vi "RF627_EXAMPLE.vi"() -> ()   [LabVIEW 2019]
doc: "This example VI calls the .NET DLL that accompanies it, which is a .NET class built in C# to emulate a very basic calculator."
uses:
  C:/Users/aagolovachev/Desktop/RLD_T14_2dScan/src/RF62X/RF62X-SDK/examples/LabVIEW/rf62Xsdk.dll
  rf62Xsdk.dll
panel:
  out "xemr":u16
  out "zmr":u16
  out "ReadParams":bool
  in  "index":i32
  in  "protocol":i32(ring)=1 items=["SERVICE_PROTOKOL"=1, "ETHERNET_IP"=2, "MODBUS_TCP"=3]
  out "Connect 2":bool
  in  "?":bool
  out "Connect":bool
  out "Count Points":i32
  out "XY Graph":cluster{"X":sgl, "Z":sgl}[](graph)
  out "Count":i32
  out "SdkInit":bool
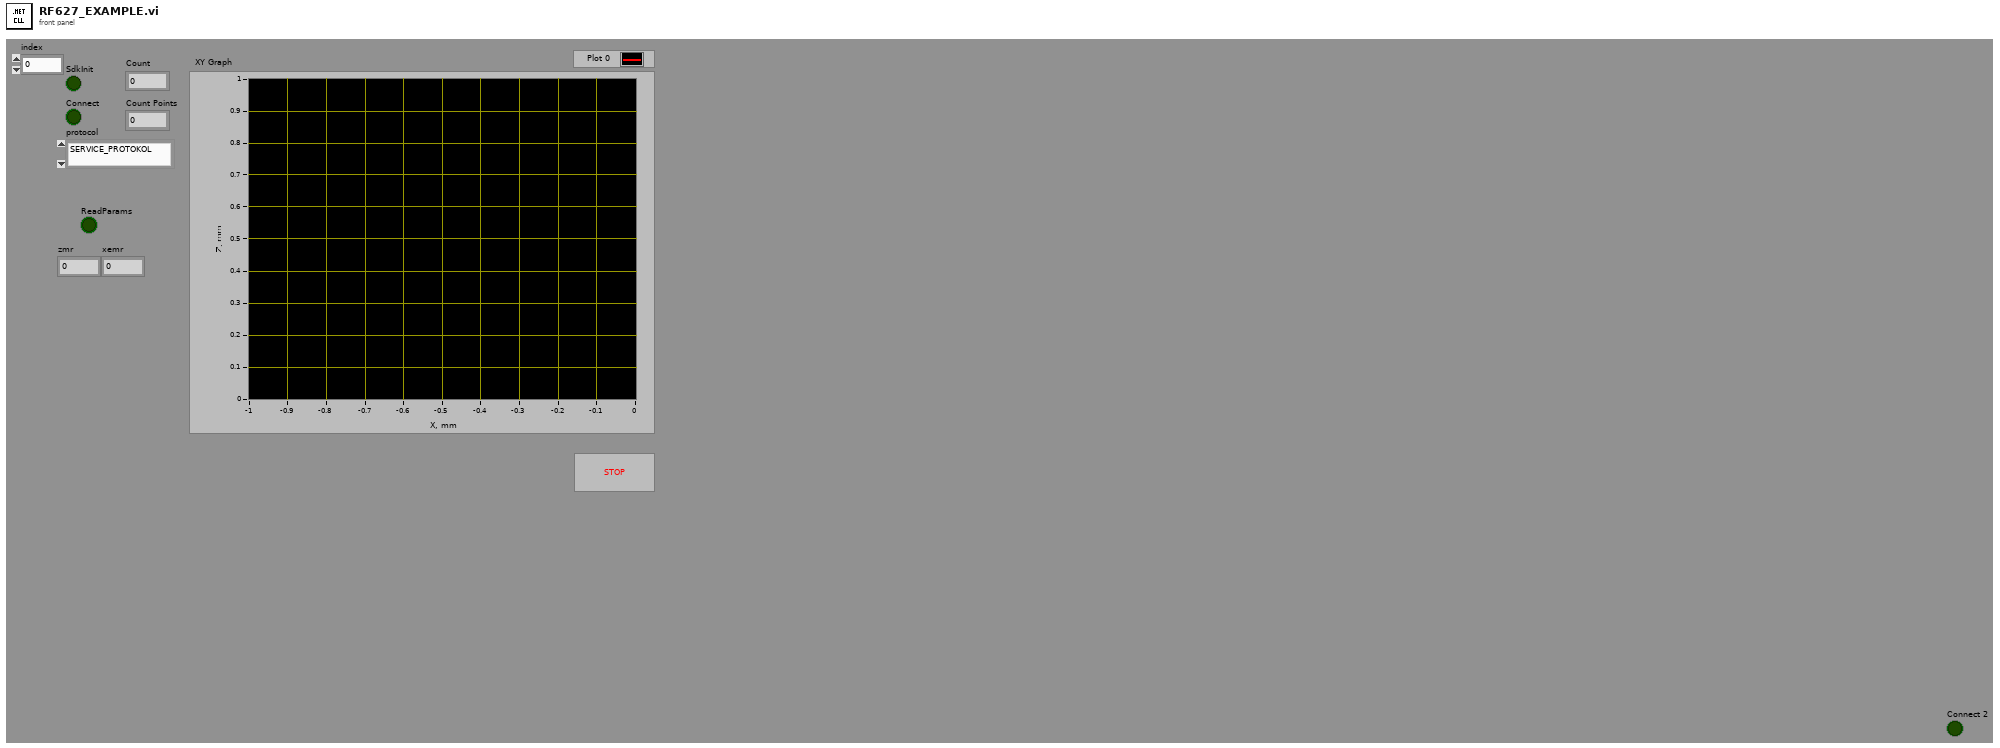
[diagram p1: front panel]
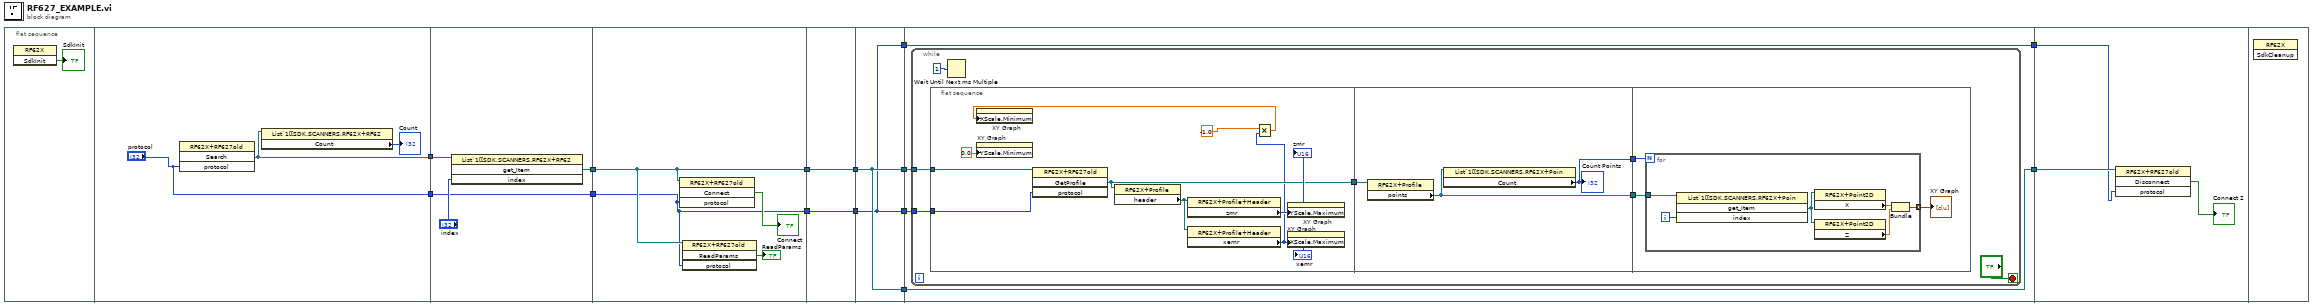
[diagram p0: block diagram]
diagram:
  n1 = flat-sequence {
    tunnel: [w17] -> w12
    tunnel: ["protocol"] -> w6
    tunnel: [w21] -> w14
    tunnel: w12 -> [w20]
    tunnel: [w19] -> w7
    tunnel: w6 -> [w19]
    tunnel: w14 -> [w25]
    tunnel: [w25] -> w13
    tunnel: w7 -> [w24]
    tunnel: [w24] -> w5
    tunnel: w13 -> [w28]
    tunnel: [w28] -> w10
    tunnel: w5 -> [w27]
    tunnel: [w27] -> w4
    tunnel: [w30] -> w11
    tunnel: w10 -> [w30]
    tunnel: [w30] -> w8
    tunnel: w4 -> [w29]
    tunnel: [w29] -> w3
    tunnel: [w29] -> w1
    tunnel: w11 -> [w34]
    tunnel: [w33] -> w9
    tunnel: w8 -> [w33]
    tunnel: w3 -> [w32]
    tunnel: [w31] -> w2
    tunnel: w1 -> [w31]
    tunnel: w9 -> [w64]
    tunnel: w2 -> [w63]
    frame #0 {
      n2 = invoke class="RF62X" method="SdkInit"() -> ("SdkInit"=→"SdkInit":bool)  [unwired: 3 in, 2 out]
    }
    frame #1 {
      n3 = invoke class="RF62X+RF627old" method="Search"("protocol"="protocol") -> ("Search"=w17:refnum<k24>)  [unwired: 3 in, 3 out]
      n4 = property class="List`1[[SDK.SCANNERS.RF62X+RF62"(reference=w17) -> ("Count"=→"Count":i32)  [unwired: 1 in, 2 out]
    }
    frame #2 {
      n5 = invoke class="List`1[[SDK.SCANNERS.RF62X+RF62" method="get_Item"(reference=w20, "index"="index") -> ("get_Item"=w21:refnum<k24>)  [unwired: 2 in, 3 out]
    }
    frame #3 {
      n6 = invoke class="RF62X+RF627old" method="Connect"(reference=w25, "protocol"=w24) -> ("Connect"=→"Connect":bool)  [unwired: 2 in, 3 out]
      n7 = invoke class="RF62X+RF627old" method="ReadParams"(reference=w25, "protocol"=w24) -> ("ReadParams"=→"ReadParams":bool)  [unwired: 2 in, 3 out]
    }
    frame #4 {
    }
    frame #5 {
    }
    frame #6 {
      n8 = while {
        tunnel: w34 -> [w39]
        tunnel: w32 -> [w35]
        stop <- "?" stop-if-true
        n9 = flat-sequence {
          tunnel: w39 -> [w50]
          tunnel: [w47] -> w38
          tunnel: w35 -> [w42]
          tunnel: w38 -> [w53]
          tunnel: [w52] -> w37
          tunnel: [w51] -> w36
          tunnel: w37 -> [w55]
          tunnel: w36 -> [w54]
          frame #0 {
            n10 = property on="XY Graph" class="XYGraph (strict)"("YScale.Minimum"=0.0 ("Y Scale.Range:Minimum")) -> ()  [unwired: 2 in, 2 out]
            n11 = invoke class="RF62X+RF627old" method="GetProfile"(reference=w50, "protocol"=w42) -> ("GetProfile"=w47:refnum<k24>)  [unwired: 2 in, 3 out]
            n12 = property class="RF62X+Profile"(reference=w47) -> ("header"=w48:refnum<k24>)  [unwired: 1 in, 2 out]
            n13 = property class="RF62X+Profile+Header"(reference=w48) -> ("zmr"=w49:u16)  [unwired: 1 in, 2 out]
            "zmr" <- w49
            n14 = property class="RF62X+Profile+Header"(reference=w48) -> ("xemr"=w44:u16)  [unwired: 1 in, 2 out]
            "xemr" <- w44
            n15 = Multiply(x=-1.0 ("Y Scale.Range:Minimum"), y=w44) -> (x*y=w43:dbl)
            n16 = property on="XY Graph" class="XYGraph (strict)"("XScale.Minimum"=w43) -> ()  [unwired: 2 in, 2 out]
            n17 = property on="XY Graph" class="XYGraph (strict)"("YScale.Maximum"=w49) -> ()  [unwired: 2 in, 2 out]
            n18 = property on="XY Graph" class="XYGraph (strict)"("XScale.Maximum"=w44) -> ()  [unwired: 2 in, 2 out]
          }
          frame #1 {
            n19 = property class="RF62X+Profile"(reference=w53) -> ("points"=w52:refnum<k24>)  [unwired: 1 in, 2 out]
            n20 = property class="List`1[[SDK.SCANNERS.RF62X+Poin"(reference=w52) -> ("Count"=w51:i32)  [unwired: 1 in, 2 out]
            "Count Points" <- w51
          }
          frame #2 {
            n21 = for {
              N: w54 -> [_]
              tunnel: [w61] -> w56 mode=indexing
              tunnel: w55 -> [w57]
              i -> [w62]
              n22 = invoke class="List`1[[SDK.SCANNERS.RF62X+Poin" method="get_Item"(reference=w57, "index"=w62) -> ("get_Item"=w60:refnum<k24>)  [unwired: 2 in, 3 out]
              n23 = property class="RF62X+Point2D"(reference=w60) -> ("X"=w59:sgl)  [unwired: 1 in, 2 out]
              n24 = property class="RF62X+Point2D"(reference=w60) -> ("Z"=w58:sgl)  [unwired: 1 in, 2 out]
              n25 = Bundle("X"=w59, "Z"=w58) -> (w61:cluster{"X":sgl, "Z":sgl})  [unwired: 1 in]
            }
            "XY Graph" <- w56
          }
        }
        n26 = Wait Until Next ms Multiple(millisecond multiple=u32 1 ("millisecond timer value")) -> ()  [unwired: 1 out]
      }
    }
    frame #7 {
      n27 = invoke class="RF62X+RF627old" method="Disconnect"(reference=w64, "protocol"=w63) -> ("Disconnect"=→"Connect 2":bool)  [unwired: 2 in, 3 out]
    }
    frame #8 {
      n28 = invoke class="RF62X" method="SdkCleanup"() -> ()  [unwired: 3 in, 3 out]
    }
  }
